vi "EV Rotator Control.vi"(0 "Run Step Inputs":T1={"Setup in"="", "Data in"=[], "Results in"=[], "Seq Setup in"="", "Step name"="", "Hardware in"="", "Calibration in"="", "Step # in sequence"=0, "Display step?(f)"=TRUE, "Generate names only"=FALSE, "Waveforms in"=[], "Memory List Grouping info"=[]} {"Waveforms in"."Y dB ref" format="%.1f"; "Waveforms in"."Y axis" items=["dB", "Lin", "Pwr"]; "Waveforms in"."Y data" items=["dB", "Lin", "Pwr"]; "Waveforms in"."X data" items=["dB", "Lin", "Pwr"]; "Data in"."Z data" items=["dB", "Lin", "Pwr"]; "Data in"."X data" items=["dB", "Lin", "Pwr"]; "Data in"."Y data" items=["dB", "Lin", "Pwr"]; "Data in"."Z dB ref" format="%.1f"; "Data in"."Z axis" items=["Log", "Lin"]; "Data in"."X dB ref" format="%.1f"; "Data in"."X axis" items=["Log", "Lin"]; "Data in"."Y axis" items=["Log", "Lin"]; "Data in"."Y dB ref" format="%.1f"; "Data in"."Curve"."z" format="%.2f"; "Data in"."Curve"."y" format="%.2f"; "Data in"."Curve"."x" format="%.2f"; "Results in"."Unit type" items=["dB", "Lin", "Pwr"]; "Results in"."Margin" format="%.2f"}, 11 "error in (no error)":errorcluster) -> (6 "Data out":T2 {"Z data" items=["dB", "Lin", "Pwr"]; "X data" items=["dB", "Lin", "Pwr"]; "Y data" items=["dB", "Lin", "Pwr"]; "Z dB ref" format="%.1f"; "Z axis" items=["Log", "Lin"]; "X dB ref" format="%.1f"; "X axis" items=["Log", "Lin"]; "Y axis" items=["Log", "Lin"]; "Y dB ref" format="%.1f"; "Curve"."z" format="%.2f"; "Curve"."y" format="%.2f"; "Curve"."x" format="%.2f"}, 8 "Results out":T5 {"Unit type" items=["dB", "Lin", "Pwr"]; "Margin" format="%.2f"}, 10 "Waveforms out":T7 {"Y dB ref" format="%.1f"; "Y axis" items=["dB", "Lin", "Pwr"]; "Y data" items=["dB", "Lin", "Pwr"]; "X data" items=["dB", "Lin", "Pwr"]}, 15 "error out":errorcluster)   [LabVIEW 2012]
uses:
  custom and SC Run Seq Sub VIs.llb/data array.ctl
  custom and SC Run Seq Sub VIs.llb/data cluster.ctl
  custom and SC Run Seq Sub VIs.llb/Axis Unit Type.ctl
  custom and SC Run Seq Sub VIs.llb/result array.ctl
  custom and SC Run Seq Sub VIs.llb/result cluster.ctl
  custom and SC Run Seq Sub VIs.llb/waveform array.ctl
  custom and SC Run Seq Sub VIs.llb/waveform cluster.ctl
  custom and SC Run Seq Sub VIs.llb/Run Step Inputs.ctl
  custom and SC Run Seq Sub VIs.llb/Memory List Grouping.ctl
  C:/SoundCheck 12.0/System/Custom VIs/EV.Rotator.RotatorControl.dll
  EV.Rotator.RotatorControl.dll
panel:
  # "NOTE:  These controls and indicators must stay here, but you can Hide them if you wish.  These are wired as the standard input/output connector pane for step run VIs."
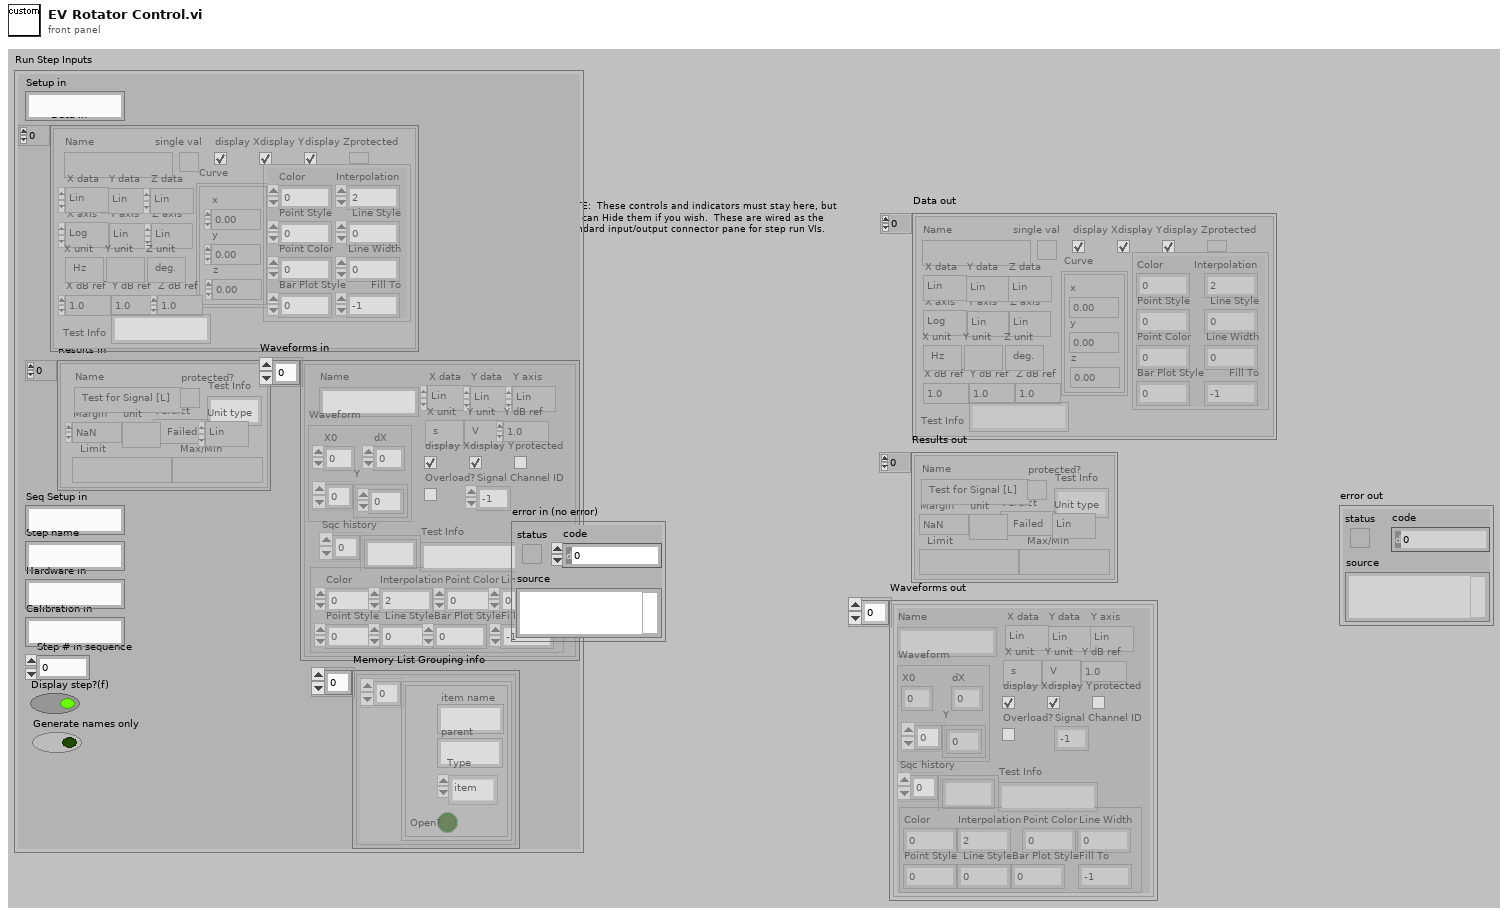
[diagram p1: front panel]
types:
  T1 = typedef "Run Step Inputs.ctl" = cluster{"Setup in":string, "Data in":T2, "Results in":T5, "Seq Setup in":string, "Step name":string, "Hardware in":string, "Calibration in":string, "Step # in sequence":i32, "Display step?(f)":bool, "Generate names only":bool, "Waveforms in":T7, "Memory List Grouping info":cluster{T9[]}[]}
  T2 = typedef "data array.ctl" = T3[]
  T3 = typedef "data cluster.ctl" = cluster{"Name":string, "Curve":cluster{"x":dbl, "y":dbl, "z":dbl}[], "X data":T4, "Y data":T4, "Z data":T4, "X axis":u16, "Y axis":u16, "Z axis":u16, "X unit":string, "Y unit":string, "Z unit":string, "X dB ref":dbl, "Y dB ref":dbl, "Z dB ref":dbl, "single val":bool, "protected":bool, "display X":bool, "display Y":bool, "display Z":bool, "Plot Settings":cluster{"Color":u32, "Interpolation":u8, "Point Style":u8, "Line Style":u8, "Point Color":u32, "Line Width":u8, "Bar Plot Style":u8, "Fill To":i16}, "Test Info":string}
  T4 = typedef "Axis Unit Type.ctl" = u16
  T5 = typedef "result array.ctl" = T6[]
  T6 = typedef "result cluster.ctl" = cluster{"Name":string, "Margin":dbl, "unit":string, "Verdict":bool, "Limit":string, "Max/Min":string, "protected?":bool, "Test Info":string, "Unit type":T4}
  T7 = typedef "waveform array.ctl" = T8[]
  T8 = typedef "waveform cluster.ctl" = cluster{"Name":string, "Waveform":cluster{"X0":dbl, "dX":dbl, "Y":sgl[]}, "X data":T4, "Y data":T4, "Y axis":T4, "X unit":string, "Y unit":string, "Y dB ref":dbl, "display Y":bool, "display X":bool, "Overload?":bool, "protected":bool, "Sqc history":string[], "Signal Channel ID":i32, "Plot Settings":cluster{"Color":u32, "Interpolation":u8, "Point Style":u8, "Line Style":u8, "Point Color":u32, "Line Width":u8, "Bar Plot Style":u8, "Fill To":i16}, "Test Info":string}
  T9 = typedef "Memory List Grouping.ctl" = cluster{"item name":string, "parent":string, "Open?":bool, "Type":enum16{"item", "custom group", "auto group"}}
  T10 = enum16{"add", "remove", "run", "clear", "vi stopped offset"}
  T11 = cluster{"Horizontal angle":dbl, "Vertical angle":dbl, "Function to run":enum16{"Home", "MoveDegrees", "EaseToEVCoords"}, "Port name":string, "Absolute position?":bool, "Dist - axis to box front":dbl}
  T12 = typedef "seq step setup.ctl" = cluster{"Input Signal Channels":i32[], "Output Signal Channels":i32[], "Curves selected":string[][], "Curves generated":string[], "Step setup flat":string, "Trigger Signal Channel":i32, "Curves Generated Assumptions":cluster{"seq-setup in":string, "Relevant subset of mem list Grouping":cluster{T9[]}[]}}
  T13 = cluster{"Curve[0]":cluster{"x":dbl, "y":dbl, "z":dbl}, "Curve[1]":cluster{"x":dbl, "y":dbl, "z":dbl}, "Curve[2]":cluster{"x":dbl, "y":dbl, "z":dbl}, "Curve[3]":cluster{"x":dbl, "y":dbl, "z":dbl}, "Curve[4]":cluster{"x":dbl, "y":dbl, "z":dbl}, "Curve[5]":cluster{"x":dbl, "y":dbl, "z":dbl}, "Curve[6]":cluster{"x":dbl, "y":dbl, "z":dbl}, "Curve[7]":cluster{"x":dbl, "y":dbl, "z":dbl}, "Curve[8]":cluster{"x":dbl, "y":dbl, "z":dbl}}
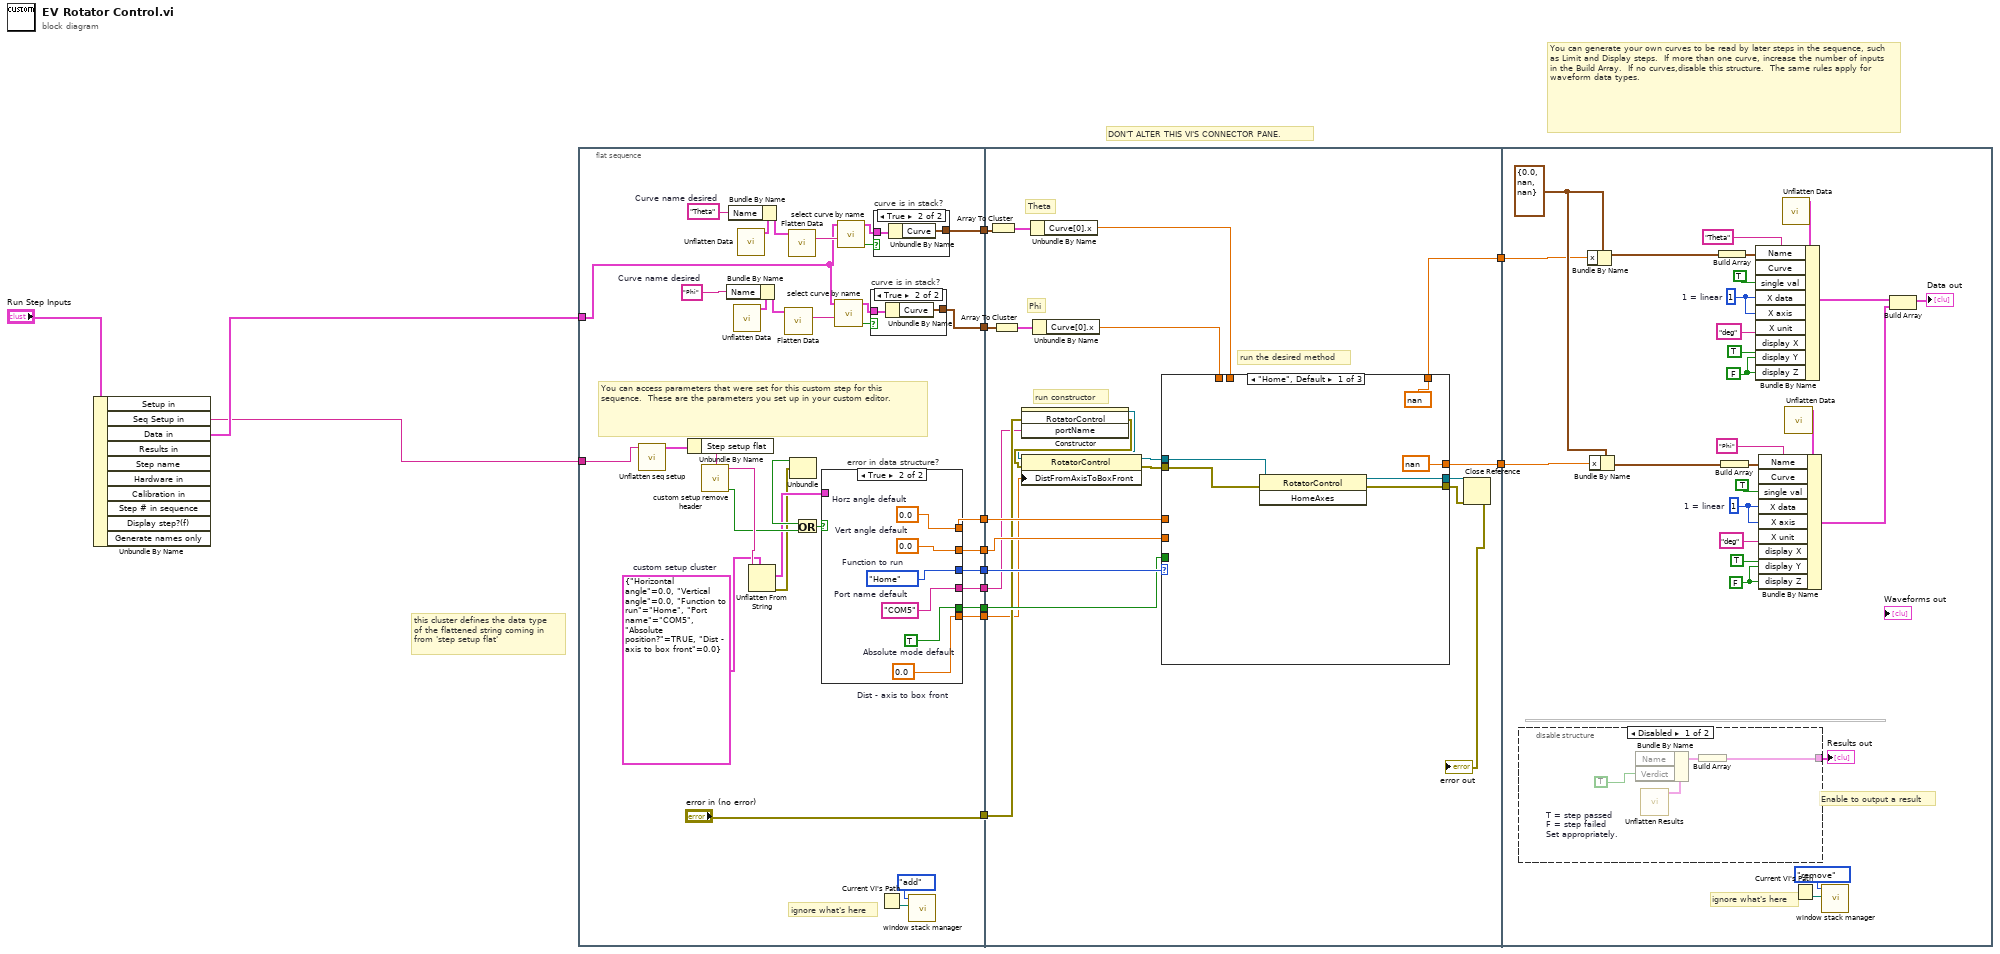
[diagram p0: block diagram]
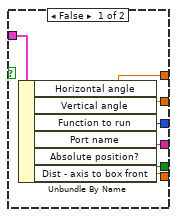
[diagram p4: hidden frame]
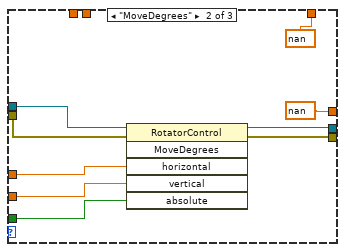
[diagram p5: hidden frame]
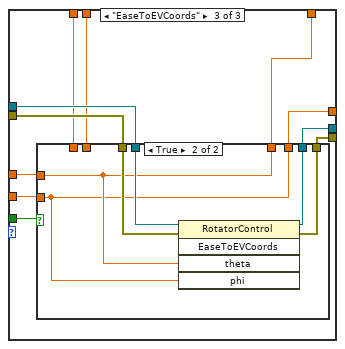
[diagram p6: hidden frame]
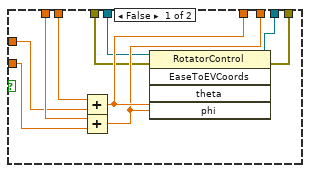
[diagram p7: hidden frame]
diagram:
  # "You can generate your own curves to be read by later steps in the sequence, such as Limit and Display steps.  If more than one curve, increase the number of inputs in the Build Array.  If no curves,disable this structure.  The same rules apply for waveform data types."
  # "this cluster defines the data type\nof the flattened string coming in\nfrom 'step setup flat'"
  # "DON'T ALTER THIS VI'S CONNECTOR PANE."
  n1 = Unbundle By Name("Run Step Inputs") -> ("Seq Setup in"=w12:string, "Data in"=w13:T2)  [unwired: 8 out]
  n2 = flat-sequence {
    tunnel: w13 -> [w17]
    tunnel: w12 -> [w37]
    tunnel: ["error in (no error)"] -> w11
    tunnel: [w35] -> w10
    tunnel: [w34] -> w9
    tunnel: [w33] -> w8
    tunnel: [w32] -> w7
    tunnel: [w31] -> w6
    tunnel: [w30] -> w5
    tunnel: [w16] -> w4
    tunnel: [w15] -> w1
    tunnel: w11 -> [w76]
    tunnel: w10 -> [w75]
    tunnel: w9 -> [w87]
    tunnel: w8 -> [w83]
    tunnel: w7 -> [w86]
    tunnel: w6 -> [w85]
    tunnel: w5 -> [w82]
    tunnel: w4 -> [w79]
    tunnel: [w74] -> w3
    tunnel: [w73] -> w2
    tunnel: w1 -> [w66]
    tunnel: w3 -> [w131]
    tunnel: w2 -> [w130]
    frame #0 {
      w20 = "Phi"  # Curve name desired
      w26 = "Theta"  # Curve name desired
      w43 = T11 {"Horizontal angle"=0.0, "Vertical angle"=0.0, "Function to run"=enum."Home", "Port name"="COM5", "Absolute position?"=TRUE, "Dist - axis to box front"=0.0}  # custom setup cluster
      # "ignore what's here"
      # "You can access parameters that were set for this custom step for this sequence.  These are the parameters you set up in your custom editor."
      n3 = call "Unflatten seq setup.vi"("Unflatten seq setup"=w37) -> ("Sequence-specific step set-up"=w48:T12)  [unwired: 3 in, 7 out]
      n4 = Unbundle By Name(w48) -> ("Step setup flat"=w47:string)
      n5 = call "custom setup remove header.vi"("Output from 'Step setup flat' of seq-setup structure"=w47) -> ("Error?"=w45:bool, "Flattened custom step setup cluster"=w46:string)  [unwired: 9 out]
      n6 = call "Unflatten Data.vi"() -> ("Datum"=w21:T3)  [unwired: 1 in, 10 out]
      n7 = Bundle By Name(cluster=w21, "Name"=w20) -> (w19:T3)
      n8 = call "Unflatten Data.vi"() -> ("Datum"=w27:T3)  [unwired: 1 in, 10 out]
      n9 = Bundle By Name(cluster=w27, "Name"=w26) -> (w25:T3)
      n10 = Unflatten From String(type=w43, binary string=w46) -> (value=w41:T11, error out=w40:errorcluster)  [unwired: 1 in, 3 out]
      n11 = call "Flatten Data.vi"("Datum"=w19) -> ("Data flattened"=w18:string)  [unwired: 10 out]
      n12 = call "Flatten Data.vi"("Datum"=w25) -> ("Data flattened"=w24:string)  [unwired: 10 out]
      n13 = Unbundle(w40) -> ("status"=w44:bool)  [unwired: 2 out]
      n14 = Or(x=w44, y=w45) -> (x .or. y?=w42:bool)
      n15 = case "error in data structure?" shown="True" w42 {
        tunnel: [w58 w65] -> w33
        tunnel: [w59 w64] -> w32
        tunnel: [w57 w61] -> w34
        tunnel: w41 -> [w56 _]
        tunnel: [w55 w63] -> w35
        tunnel: [w54 w62] -> w31
        tunnel: [w53 w60] -> w15
        frame False {
          n16 = Unbundle By Name(w56) -> ("Horizontal angle"=w58:dbl, "Vertical angle"=w59:dbl, "Function to run"=w57:enum16{"Home", "MoveDegrees", "EaseToEVCoords"}, "Port name"=w55:string, "Absolute position?"=w54:bool, "Dist - axis to box front"=w53:dbl)
        }
        frame True {
          w60 = 0.0  # Dist - axis to box front
          w61 = enum16{"Home", "MoveDegrees", "EaseToEVCoords"}."Home"  # Function to run
          w62 = TRUE  # Absolute mode default
          w63 = "COM5"  # Port name default
          w64 = 0.0  # Vert angle default
          w65 = 0.0  # Horz angle default
        }
      }
      n17 = call "select curve by name.vi"("Curve name desired (flat data)"=w18, "Data array in"=w17) -> ("Exists?"=w23:bool, "Desired curve"=w22:T3)  [unwired: 1 in, 7 out]
      n18 = call "select curve by name.vi"("Curve name desired (flat data)"=w24, "Data array in"=w17) -> ("Exists?"=w29:bool, "Desired curve"=w28:T3)  [unwired: 1 in, 7 out]
      n19 = case "curve is in stack?" shown="True" w23 {
        tunnel: w22 -> [_ w50]
        tunnel: [_ w49] -> w16
        frame False {
        }
        frame True {
          n20 = Unbundle By Name(w50) -> ("Curve"=w49:cluster{"x":dbl, "y":dbl, "z":dbl}[])
        }
      }
      n21 = case "curve is in stack?" shown="True" w29 {
        tunnel: w28 -> [_ w52]
        tunnel: [_ w51] -> w30
        frame False {
        }
        frame True {
          n22 = Unbundle By Name(w52) -> ("Curve"=w51:cluster{"x":dbl, "y":dbl, "z":dbl}[])
        }
      }
      n23 = Current VI's Path() -> (path=w39:path)
      n24 = call "window stack manager.vi"("VI path"=w39, "Function (run)"=T10."add") -> ()  [unwired: 5 in, 5 out]
    }
    frame #1 {
      # "run the desired method"
      # "run constructor"
      # "Theta"
      # "Phi"
      n25 = Array To Cluster(array=w82) -> (cluster=w81:T13)
      n26 = Array To Cluster(array=w79) -> (cluster=w80:T13)
      n27 = constructor class="RotatorControl"(error in=w76, "portName"=w75) -> (reference out=w69:refnum<k24>, error out=w70:errorcluster)  [unwired: 2 in, 2 out]
      n28 = property class="RotatorControl"(reference=w69, error in=w70, "DistFromAxisToBoxFront"=w66) -> (reference out=w68:refnum<k24>, error out=w67:errorcluster)
      n29 = Unbundle By Name(w81) -> ("Curve[0].x"=w72:dbl)
      n30 = Unbundle By Name(w80) -> ("Curve[0].x"=w71:dbl)
      n31 = case shown="\"Home\", Default" w87 {
        tunnel: w68 -> [w92 w102 w113]
        tunnel: w83 -> [_ w101 w109]
        tunnel: w86 -> [_ w100 w108]
        tunnel: w85 -> [_ w99 w107]
        tunnel: w67 -> [w93 w96 w112]
        tunnel: [w91 w98 w111] -> w78
        tunnel: [w90 w97 w110] -> w77
        tunnel: [nan ("Horz angle default") nan ("Horz angle default") w106] -> w74
        tunnel: [nan ("Horz angle default") nan ("Horz angle default") w105] -> w73
        tunnel: w72 -> [_ _ w104]
        tunnel: w71 -> [_ _ w103]
        frame "Home", Default {
          n32 = invoke class="RotatorControl" method="HomeAxes"(reference=w92, error in=w93) -> (reference out=w90:refnum<k24>, error out=w91:errorcluster)  [unwired: 1 in, 1 out]
        }
        frame "MoveDegrees" {
          n33 = invoke class="RotatorControl" method="MoveDegrees"(reference=w102, error in=w96, "horizontal"=w101, "vertical"=w100, "absolute"=w99) -> (reference out=w97:refnum<k24>, error out=w98:errorcluster)  [unwired: 1 in, 4 out]
        }
        frame "EaseToEVCoords" {
          n34 = case shown="True" w107 {
            tunnel: w113 -> [w115 w129]
            tunnel: w112 -> [w114 w128]
            tunnel: [w122 w127] -> w111
            tunnel: [w123 w126] -> w110
            tunnel: w109 -> [w117 w125]
            tunnel: w108 -> [w119 w124]
            tunnel: [w121 w125] -> w106
            tunnel: [w120 w124] -> w105
            tunnel: w104 -> [w116 _]
            tunnel: w103 -> [w118 _]
            frame False {
              n35 = Add(x=w116, y=w117) -> (x+y=w121:dbl)
              n36 = Add(x=w118, y=w119) -> (x+y=w120:dbl)
              n37 = invoke class="RotatorControl" method="EaseToEVCoords"(reference=w115, error in=w114, "theta"=w121, "phi"=w120) -> (reference out=w123:refnum<k24>, error out=w122:errorcluster)  [unwired: 1 in, 3 out]
            }
            frame True {
              n38 = invoke class="RotatorControl" method="EaseToEVCoords"(reference=w129, error in=w128, "theta"=w125, "phi"=w124) -> (reference out=w126:refnum<k24>, error out=w127:errorcluster)  [unwired: 1 in, 3 out]
            }
          }
        }
      }
      n39 = Close Reference(reference=w77, error in (no error)=w78) -> (error out=→"error out":errorcluster)
    }
    frame #2 {
      w135 = FALSE ("display Y")
      w134 = u16 1  # 1 = linear
      w144 = FALSE ("display Y")
      w133 = cluster{"x":dbl, "y":dbl, "z":dbl} {"x"=0.0, "y"=nan, "z"=nan}
      w143 = u16 1  # 1 = linear
      # "ignore what's here"
      # "Enable to output a result"
      n40 = disable-structure shown="Disabled" {
        disable-tunnel: [w160 _] -> w155
        frame Disabled {
          w158 = TRUE  # T = step passed F = step failed Set appropriately.
          n41 = call "Unflatten Results.vi"() -> ("Result"=w157:T6)  [unwired: 1 in, 10 out]
          n42 = Bundle By Name(cluster=w157, "Verdict"=w158) -> (w159:T6)  [unwired: 1 in]
          n43 = Build Array(w159) -> (w160:T6[])
        }
        frame Enabled {
          # "This whole \"Results out\" structure is mandatory."
        }
      }
      "Results out" <- w155
      n44 = Bundle By Name(cluster=w133, "x"=w131) -> (w149:cluster{"x":dbl, "y":dbl, "z":dbl})
      n45 = Bundle By Name(cluster=w133, "x"=w130) -> (w140:cluster{"x":dbl, "y":dbl, "z":dbl})
      n46 = Build Array(w149) -> (w148:cluster{"x":dbl, "y":dbl, "z":dbl}[])
      n47 = Build Array(w140) -> (w139:cluster{"x":dbl, "y":dbl, "z":dbl}[])
      n48 = call "Unflatten Data.vi"() -> ("Datum"=w150:T3)  [unwired: 1 in, 10 out]
      n49 = Bundle By Name(cluster=w150, "Name"="Theta" ("Bundle Element"), "Curve"=w148, "single val"=TRUE ("T = data is just a single number (the Y element)"), "X data"=w143, "X axis"=w143, "X unit"="deg", "display X"=TRUE, "display Y"=w144, "display Z"=w144) -> (w152:T3)
      n50 = call "Unflatten Data.vi"() -> ("Datum"=w141:T3)  [unwired: 1 in, 10 out]
      n51 = Bundle By Name(cluster=w141, "Name"="Phi" ("Bundle Element"), "Curve"=w139, "single val"=TRUE ("T = data is just a single number (the Y element)"), "X data"=w134, "X axis"=w134, "X unit"="deg", "display X"=TRUE, "display Y"=w135, "display Z"=w135) -> (w132:T3)
      n52 = Current VI's Path() -> (path=w153:path)
      n53 = call "window stack manager.vi"("VI path"=w153, "Function (run)"=enum16{"add", "remove", "run", "clear"}."remove") -> ()  [unwired: 5 in, 5 out]
      n54 = Build Array(w152, w132) -> (→"Data out":T3[])
    }
  }
